vi "Read Legend Position.vi"(9 "WaveformChart in":refnum<class "WaveformGraph.lvclass">) -> (3 "WaveformChart out":refnum<class "WaveformGraph.lvclass">, 4 "Legend Position":cluster{"Left":i32, "Top":i32})   [LabVIEW 2014, in "WaveformGraph.lvclass"]
uses:
  WaveformGraph.lvclass
  WaveformGraph.lvclass/WaveformGraph.ctl
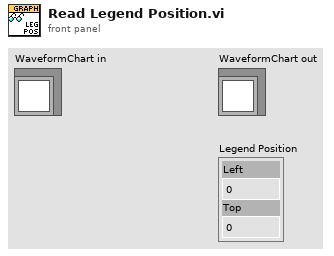
[diagram p1: front panel]
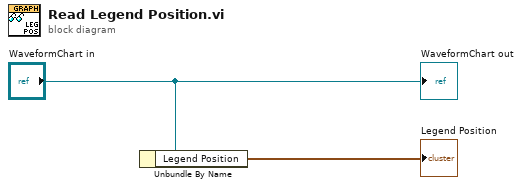
[diagram p0: block diagram]
diagram:
  n1 = Unbundle By Name("WaveformChart in") -> ("Legend Position"=→"Legend Position":cluster{"Left":i32, "Top":i32})
  "WaveformChart out" <- "WaveformChart in"
